vi "Set Lift PID.vi"(11 "setpoint":dbl format="%.2f") -> ()   [LabVIEW 2015]
uses:
  <vilib>/addons/control/pid/pid.llb/PID (DBL).vi
  <vilib>/addons/control/pid/NI_PID_pid.lvlib
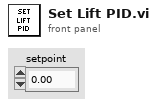
[diagram p1: front panel]
types:
  T1 = cluster{"proportional gain (Kc)":dbl, "integral time (Ti, min)":dbl, "derivative time (Td, min)":dbl}
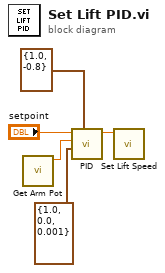
[diagram p0: block diagram]
diagram:
  n1 = call "Get Arm Pot.vi"() -> ("Normalized Value"=w3:dbl)  [unwired: 11 in]
  n2 = call-poly <vilib>:"PID.vi"("output range"=cluster{"output high":dbl, "output low":dbl} {"output high"=1.0, "output low"=-0.8}, "PID gains"=T1 {"proportional gain (Kc)"=1.0, "integral time (Ti, min)"=0.0, "derivative time (Td, min)"=0.001}, "process variable"=w3, "setpoint"="setpoint") -> ("output"=w1:dbl)  [unwired: 6 in, 1 out]
  n3 = call "Set Lift Speed.vi"("Speed"=w1) -> ()  [unwired: 11 in]
